vi "No Joystick.vi"(10 "Input":variant, 11 "Data in":waveform(dbl)[](array[waveform])) -> (1 "Incorrect movement":bool, 2 "Correct movement":bool, 3 "Centered":bool)   [LabVIEW 2010]
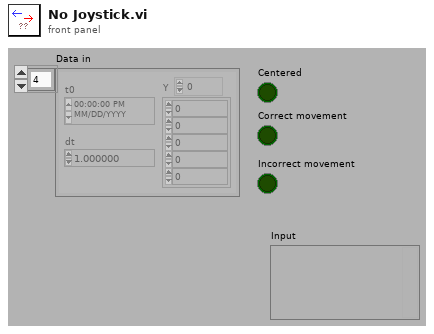
[diagram p1: front panel]
types:
  T1 = cluster{"Trial Type":i32, "Joystick Threshold":dbl, "Fixation Radius":dbl}
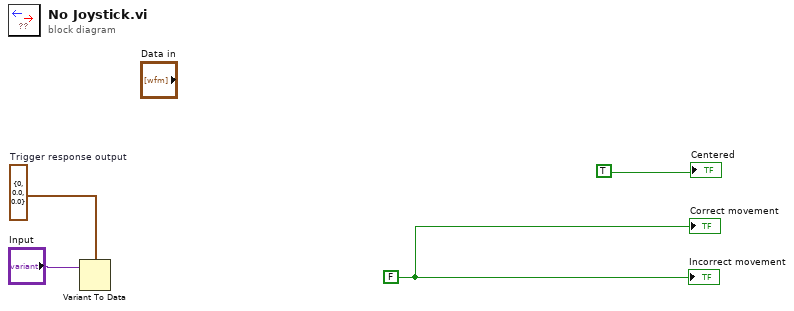
[diagram p0: block diagram]
diagram:
  w1 = FALSE
  w3 = T1 {"Trial Type"=0, "Joystick Threshold"=0.0, "Fixation Radius"=0.0}  # Trigger response output
  n1 = Variant To Data(Variant="Input", type=w3) -> ()  [unwired: 1 in, 2 out]
  "Centered" <- TRUE
  "Correct movement" <- w1
  "Incorrect movement" <- w1
